vi "Go to Voice.vi"(8 "error in (no error)":errorcluster, 11 "Voice in":refnum<class "Voice.lvclass">) -> (0 "error out":errorcluster, 3 "Process State out":refnum<class "State Actor.lvclass">)   [LabVIEW 2014, in "Voice.lvclass"]
doc: "This override disables the entry behavior when transitioning to the Running state."
uses:
  Voice.lvclass
  <vilib>/NI/Actors/State Actor/State Actor/State Actor.lvclass
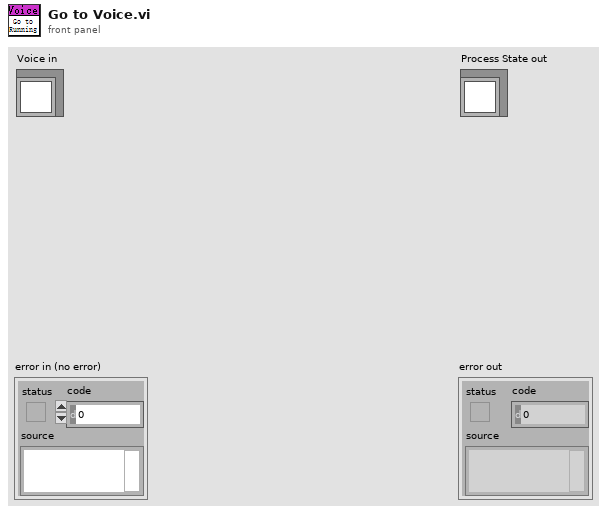
[diagram p1: front panel]
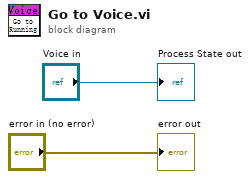
[diagram p0: block diagram]
diagram:
  "error out" <- "error in (no error)"
  "Process State out" <- "Voice in"
